vi "updateWaypoints.vi"(8 "error in (no error)":errorcluster, 11 "Drive in":refnum<class "DriveTo.lvclass">) -> (0 "error out":errorcluster, 3 "Drive out":refnum<class "DriveTo.lvclass">)   [LabVIEW 2011, in "DriveTo.lvclass"]
uses:
  DriveTo.lvclass
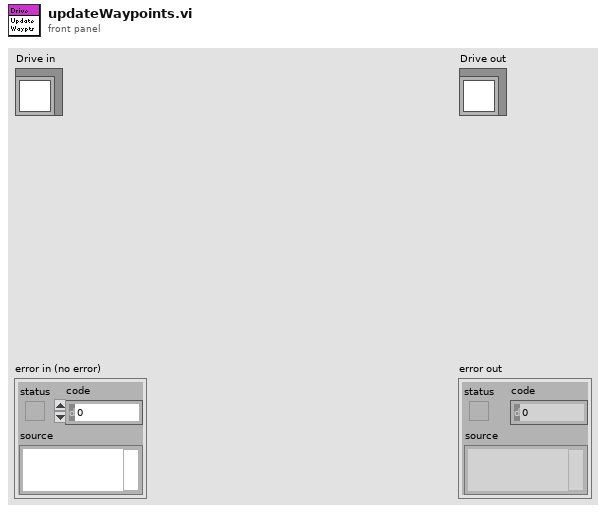
[diagram p1: front panel]
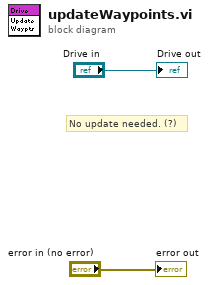
[diagram p0: block diagram]
diagram:
  # "No update needed. (?)"
  "error out" <- "error in (no error)"
  "Drive out" <- "Drive in"
